vi "LcWebView_AlertDialog_Example.vi"() -> ()   [LabVIEW 2018, in "LcWebView.lvclass"]
doc: "Inject javascript arguments"
uses:
  LcWebView.lvclass
  C:/Users/ziggz/OneDrive/Documents/GitHub/LcWebView2/LcWebView/data/Microsoft.Web.WebView2.WinForms.dll
  Documents/GitHub/LcWebView2/LcWebView/data/Microsoft.Web.WebView2.WinForms.dll
panel:
  out "BrowserProcessId":u32
  out "Status Message":string
  in  "stop":bool
  in  "Web":refnum<k24>(container)
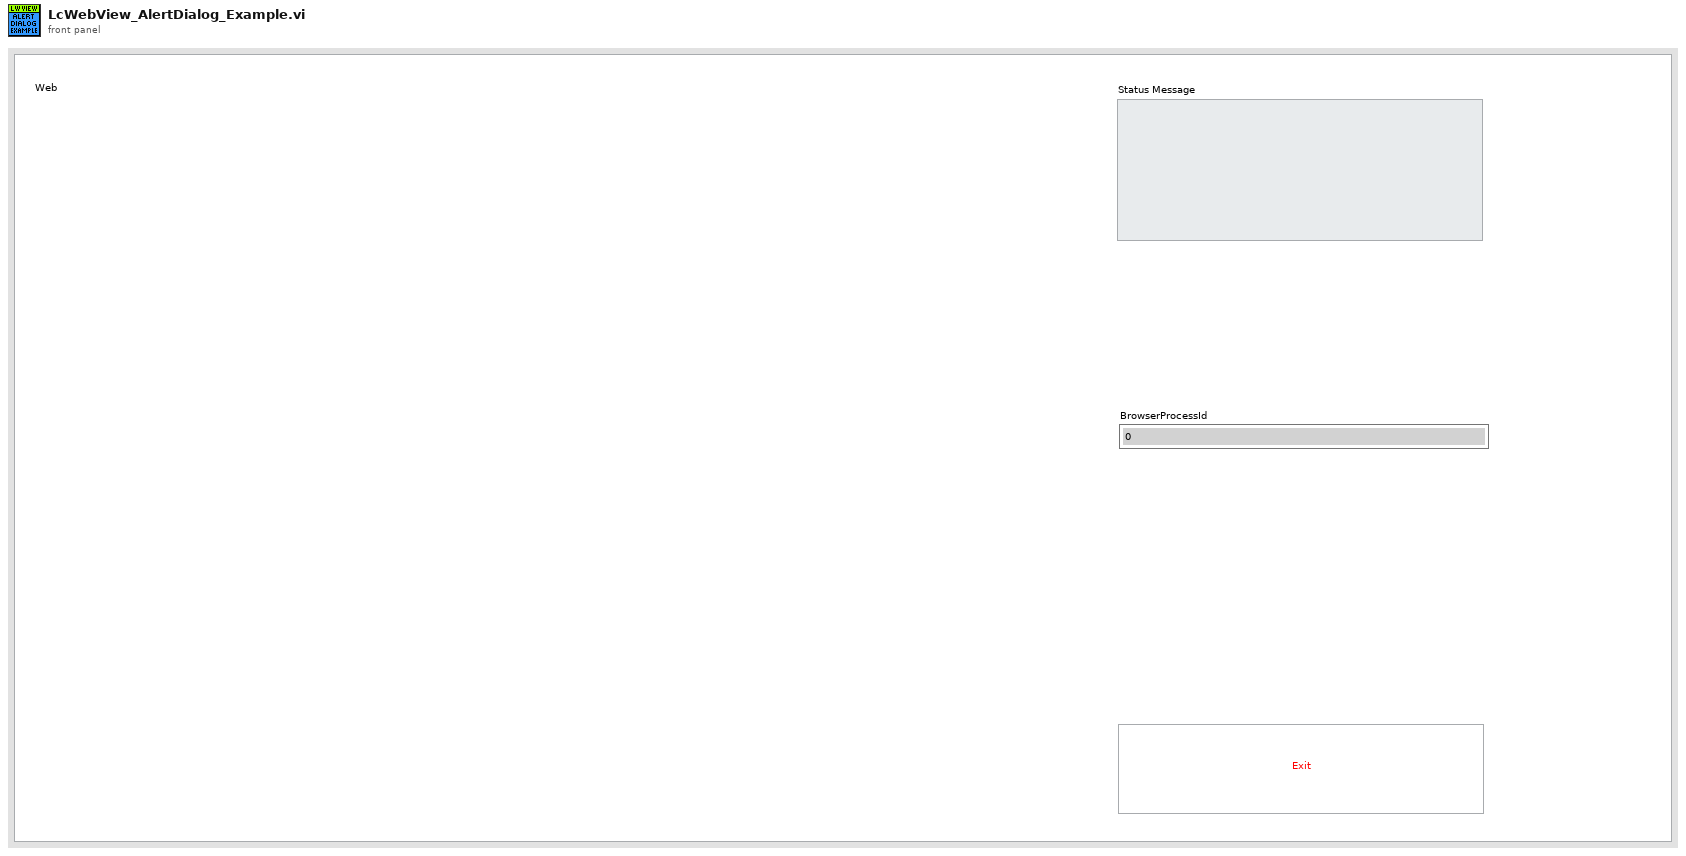
[diagram p1: front panel]
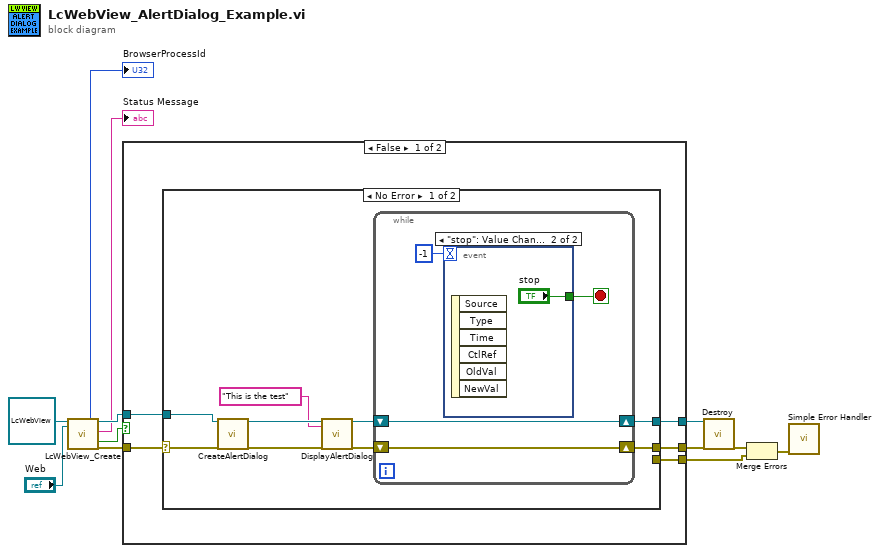
[diagram p0: block diagram]
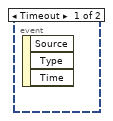
[diagram p2: hidden frame]
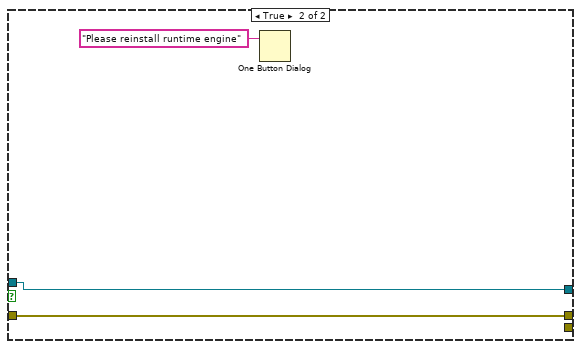
[diagram p4: hidden frame]
diagram:
  n1 = call "LcWebView_Create.vi"("reference in"=refnum<class "LcWebView.lvclass"> refnum, "Webview container"="Web") -> ("BrowserProcessId"=→"BrowserProcessId":u32, "reference out"=w10:refnum<class "LcWebView.lvclass">, "Status Message"=→"Status Message":string, "Reinstall Runtime"=w3:bool, "Error Out"=w9:errorcluster)  [unwired: 10 in, 3 out]
  n2 = case shown="False" w3 {
    tunnel: w10 -> [w17 w36]
    tunnel: w9 -> [w16 w35]
    tunnel: [w15 w36] -> w8
    tunnel: [w13 w35] -> w7
    tunnel: [w14 _] -> w4
    frame False {
      n3 = case shown="No Error" w16 {
        selector: w16 -> [w23 w32]
        tunnel: w17 -> [w24 w33]
        tunnel: [w25 w33] -> w15
        tunnel: [w26 _] -> w13
        tunnel: [_ w32] -> w14
        frame No Error {
          n4 = call-dynamic "CreateAlertDialog.vi"("reference in"=w24, "Error In"=w23) -> ("reference out"=w22:refnum<class "LcWebView.lvclass">, "Error Out"=w21:errorcluster)  [unwired: 16 in]
          n5 = call-dynamic "DisplayAlertDialog.vi"("reference in"=w22, "Message"="This is the test" ("Status Message"), "Error In"=w21) -> ("reference out"=w20:refnum<class "LcWebView.lvclass">, "Error Out"=w19:errorcluster)  [unwired: 15 in]
          n6 = while {
            shift-right: [w30] -> w25
            shift-left: w20 -> [w30]
            shift-right: [w29] -> w26
            shift-left: w19 -> [w29]
            stop <- w27 stop-if-true
            n7 = event shown="[1] \"stop\": Value Change" {
              selector: _ -> [_ _]
              dyn-events: _ -> [_ _]
              timeout: -1 -> [_ _]
              tunnel: [_ "stop"] -> w27
              event Timeout {
                n8 = event-data() -> ()  [unwired: 1 in, 3 out]
              }
              event "stop": Value Change {
                n9 = event-data() -> ()  [unwired: 1 in, 6 out]
              }
            }
          }
        }
        frame Error {
        }
      }
    }
    frame True {
      n10 = One Button Dialog(message="Please reinstall runtime engine") -> ()  [unwired: 1 in, 1 out]
    }
  }
  n11 = call-dynamic "Destroy.vi"("reference in"=w8, "Error In"=w7) -> ("Error Out"=w6:errorcluster)  [unwired: 16 in, 1 out]
  n12 = Merge Errors(w6, w4) -> (w1:errorcluster)
  n13 = call <vilib>:"Simple Error Handler.vi"("error in (no error)"=w1) -> ()  [unwired: 4 in, 5 out]
